vi "Add Datasets.vi"(8 "error in (no error)":errorcluster, 9 "Dataset Variant":variant, 10 "Datasets":T1[](array[typedef]), 11 "CubeLogger in":refnum<class "CubeLogger.lvclass">) -> (0 "error out":errorcluster, 2 "Incomplete?":bool, 3 "CubeLogger out":refnum<class "CubeLogger.lvclass">)   [LabVIEW 2018, in "CubeLogger.lvclass"]
uses:
  CubeLogger.lvclass
  Dataset.ctl
  CubeLogger.lvclass/CubeLogger.ctl
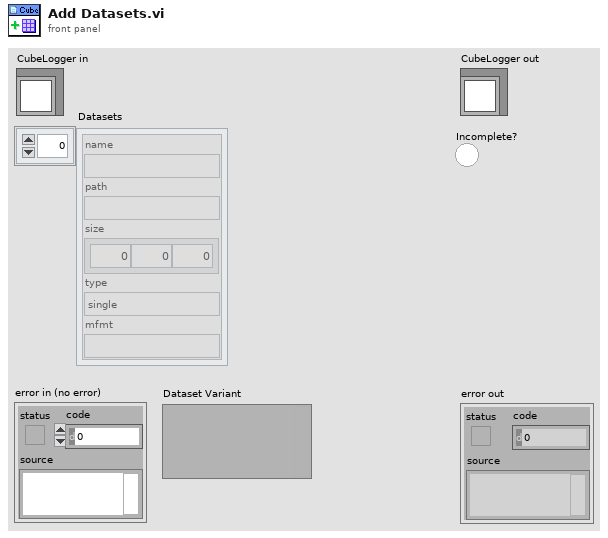
[diagram p1: front panel]
types:
  T1 = typedef "CubeLogger.lvclass/Dataset.ctl" = cluster{"name":string, "path":string, "size":i32[], "type":enum16{"single", "double", "uint8", "uint16", "uint32", "uint64", "int8", "int16", "int32", "int64"}, "mfmt":string}
  T2 = typedef "CubeLogger.lvclass/Endianness.ctl" = enum16{"big-endian, network order", "native, host order", "little-endian"}
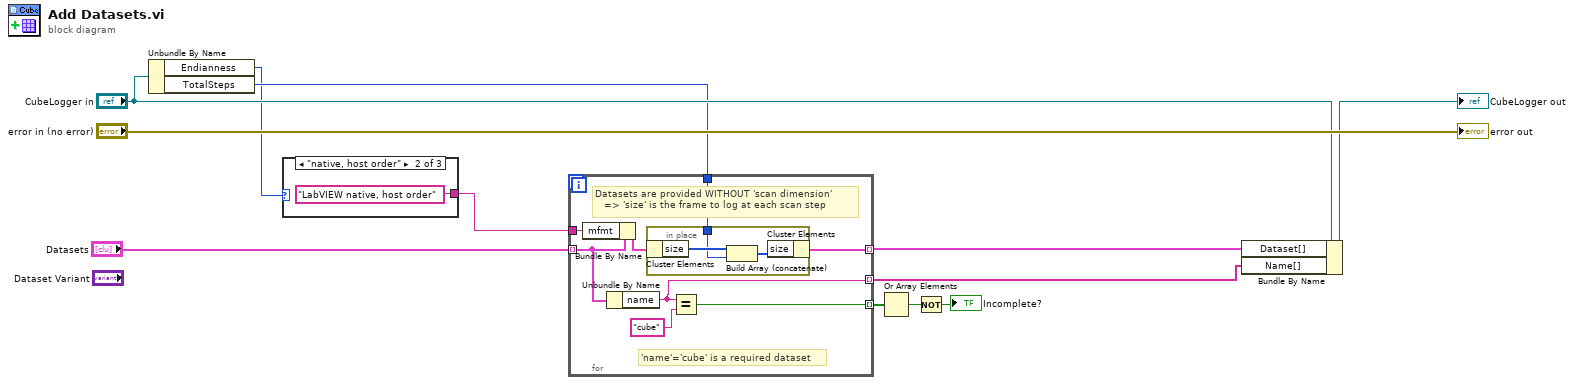
[diagram p0: block diagram]
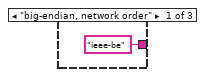
[diagram p2: hidden frame]
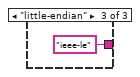
[diagram p3: hidden frame]
diagram:
  n1 = Unbundle By Name("CubeLogger in") -> ("Endianness"=w3:T2, "TotalSteps"=w9:i32)
  n2 = case shown="\"native, host order\"" w3 {
    tunnel: ["ieee-be" "LabVIEW native, host order" "ieee-le"] -> w2
    frame "big-endian, network order" {
    }
    frame "native, host order" {
    }
    frame "little-endian" {
    }
  }
  n3 = for {
    tunnel: "Datasets" -> [w21] mode=indexing
    tunnel: w9 -> [w23]
    tunnel: [w22] -> w1 mode=indexing
    tunnel: [w19] -> w7 mode=indexing
    tunnel: [w18] -> w4 mode=indexing
    tunnel: w2 -> [w16]
    # "'name'='cube' is a required dataset"
    # "Datasets are provided WITHOUT 'scan dimension'\n   => 'size' is the frame to log at each scan step"
    n4 = Bundle By Name(cluster=w21, "mfmt"=w16) -> (w17:T1)
    n5 = Unbundle By Name(w21) -> ("name"=w18:string)
    n6 = in-place {
      in-place-border: w23 -> [w24]
      n7 = in-place-cluster #1(w17) -> ("size"=w26:i32[])
      n8 = Build Array (concatenate)(w26, w24) -> (w25:i32[])
      n9 = in-place-cluster #1("size"=w25) -> (w22:T1)
    }
    n10 = Equal?(x=w18, y="cube") -> (x = y?=w19:bool)
  }
  n11 = Or Array Elements(Boolean array=w7) -> (logical OR=w6:bool)
  n12 = Not(x=w6) -> (.not. x?=→"Incomplete?":bool)
  n13 = Bundle By Name(cluster="CubeLogger in", "Dataset[]"=w1, "Name[]"=w4) -> (→"CubeLogger out":refnum<class "CubeLogger.lvclass">)
  "error out" <- "error in (no error)"
